vi "Error Handling.vi"(6 "Error String":string, 8 "Error Code":i32, 9 "Error In":errorcluster) -> (1 "Error Out":errorcluster)   [LabVIEW 2022 SP3]
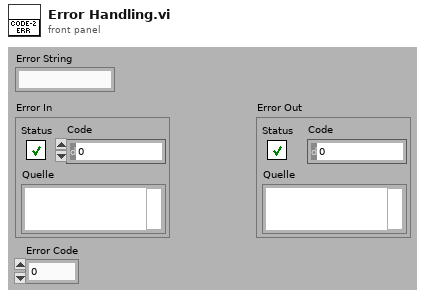
[diagram p1: front panel]
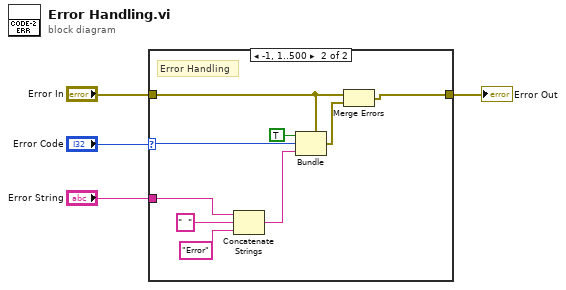
[diagram p0: block diagram]
diagram:
  n1 = case shown="-1, 1..500" "Error Code" {
    selector: "Error Code" -> [_ w9]
    tunnel: "Error In" -> [w5 w7]
    tunnel: [w5 w6] -> w3
    tunnel: "Error String" -> [_ w10]
    frame 0, Default {
      # "Error Handling"
    }
    frame -1, 1..500 {
      # "Error Handling"
      n2 = Concatenate Strings(w10, "  ", "Error") -> (w13:string)
      n3 = Bundle(cluster=w7, "status"=TRUE, "code"=w9, "source"=w13) -> (w8:errorcluster)
      n4 = Merge Errors(w7, w8) -> (w6:errorcluster)
    }
  }
  "Error Out" <- w3
